vi "Read Message.vi"(8 "error in (no error)":errorcluster, 11 "RemoteControl.ZMQ in":refnum<class "RemoteControl.ZMQ.lvclass">) -> (0 "error out":errorcluster, 1 "Data":string, 2 "Command":string, 3 "RemoteControl.ZMQ out":refnum<class "RemoteControl.ZMQ.lvclass">, 4 "ID":string)   [LabVIEW 2019, in "RemoteControl.ZMQ.lvlib" / "RemoteControl.ZMQ.lvclass"]
uses:
  RemoteControl.ZMQ.lvclass
  <vilib>/addons/zeromq/zmq_socket.lvclass
  <vilib>/addons/zeromq/zmq_context.lvclass
  <vilib>/Utility/error.llb/Error Cluster From Error Code.vi
  <vilib>/ErrorRing/Error Ring.xnode
  <vilib>/PRIrvin/JSON-RPC/JSON-RPC.lvlib
  <userlib>/LevyLab/RemoteControl/RemoteControl/RemoteControl.lvclass
  C:/Program Files (x86)/National Instruments/LabVIEW 2019/user.lib/LevyLab/RemoteControl/RemoteControl/RemoteControl.lvclass
  C:/Program Files (x86)/National Instruments/LabVIEW 2019/vi.lib/JKI/JKI SMO/smo.lvlibp/SMO/SMO.lvclass
panel:
  out "Retry#":i32
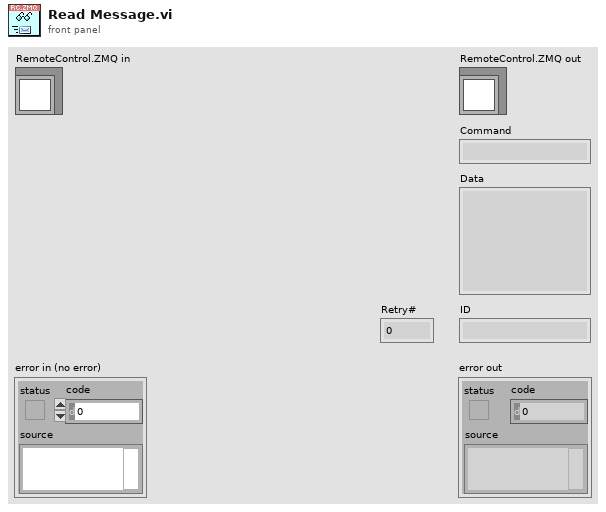
[diagram p1: front panel]
types:
  T1 = typedef "zeromq.lvlib/socket_type.ctl" = enum8{"ZMQ_PAIR", "ZMQ_PUB", "ZMQ_SUB", "ZMQ_REQ", "ZMQ_REP", "ZMQ_DEALER", "ZMQ_ROUTER", "ZMQ_PULL", "ZMQ_PUSH", "ZMQ_XPUB", "ZMQ_XSUB", "ZMQ_STREAM", "ZMQ_SERVER", "ZMQ_CLIENT", "ZMQ_RADIO", "ZMQ_DISH", "ZMQ_GATHER", "ZMQ_SCATTER", "ZMQ_DGRAM"}
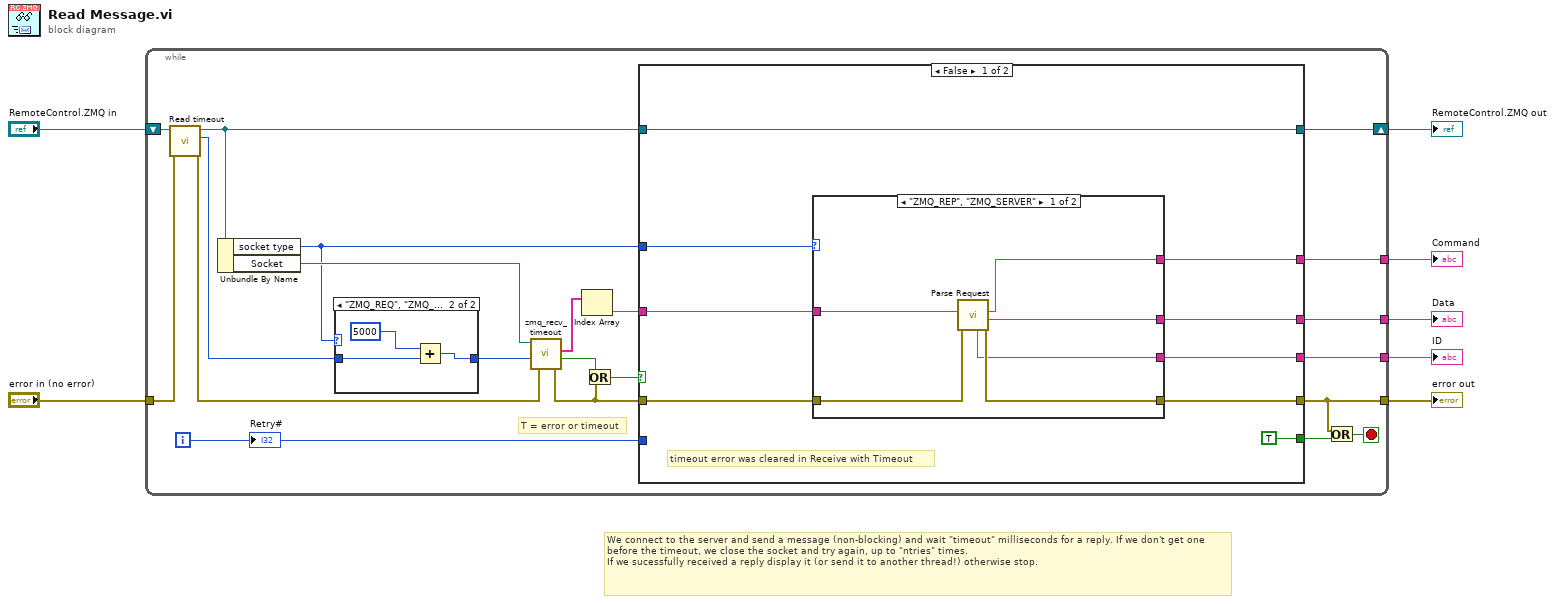
[diagram p0: block diagram]
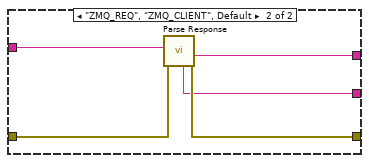
[diagram p3: hidden frame]
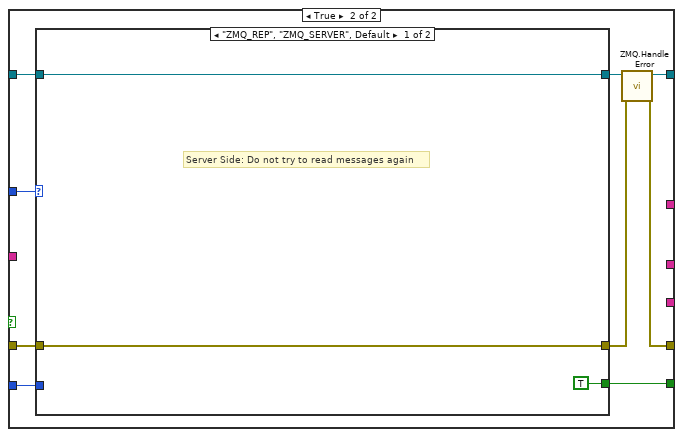
[diagram p4: hidden frame]
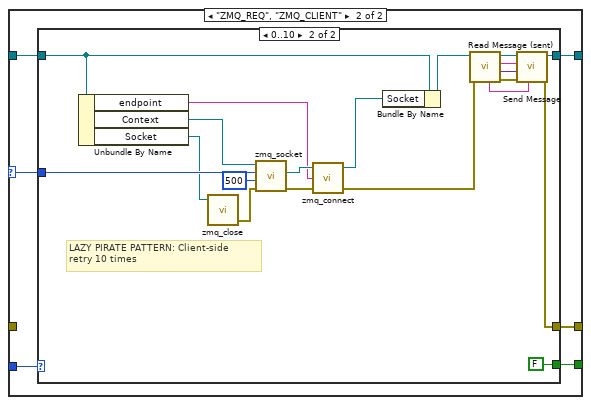
[diagram p5: hidden frame]
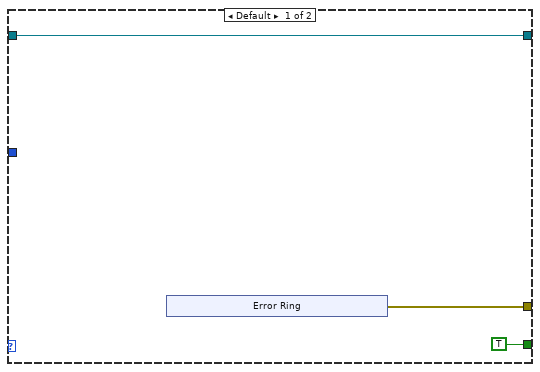
[diagram p6: hidden frame]
diagram:
  # "We connect to the server and send a message (non-blocking) and wait \"timeout\" milliseconds for a reply. If we don't get one before the timeout, we close the socket and try again, up to \"ntries\" times.\nIf we sucessfully received a reply display it (or send it to another thread!) otherwise stop."
  n1 = while {
    tunnel: [w28] -> w7
    tunnel: [w27] -> w6
    tunnel: [w26] -> w5
    tunnel: "error in (no error)" -> [w11]
    tunnel: [w14] -> w4
    shift-right: [w13] -> w3
    shift-left: "RemoteControl.ZMQ in" -> [w12]
    i -> [w23]
    stop <- w25 stop-if-true
    # "T = error or timeout"
    n2 = call <userlib>:"Read timeout.vi"("error in (no error)"=w11, "RemoteControl in"=w12) -> ("error out"=w17:errorcluster, "timeout"=w9:i32, "RemoteControl out"=w16:refnum<class "RemoteControl.ZMQ.lvclass">)  [unwired: 7 in]
    n3 = Unbundle By Name(w16) -> ("socket type"=w10:T1, "Socket"=w18:refnum<class "zmq_socket.lvclass">)
    n4 = case shown="\"ZMQ_REQ\", \"ZMQ_CLIENT\"" w10 {
      tunnel: w9 -> [w29 w32]
      tunnel: [w29 w31] -> w8
      frame "ZMQ_REP", "ZMQ_SERVER", Default {
      }
      frame "ZMQ_REQ", "ZMQ_CLIENT" {
        n5 = Add(x=5000, y=w32) -> (x+y=w31:i32)
      }
    }
    n6 = call <vilib>:"zmq_recv_timeout.vi"("error in"=w17, "timeout (ms)"=w8, "socket in"=w18) -> ("error out"=w21:errorcluster, "timeout?"=w20:bool, "parts"=w15:string[])  [unwired: 1 in, 1 out]
    n7 = Index Array(array=w15) -> (element=w22:string)  [unwired: 1 in]
    n8 = Or(x=w20, y=w21) -> (x .or. y?=w19:bool)
    n9 = case shown="False" w19 {
      tunnel: [w41 _] -> w27
      tunnel: [w40 _] -> w26
      tunnel: [w39 _] -> w28
      tunnel: w10 -> [w38 w60]
      tunnel: w16 -> [w37 w61]
      tunnel: [w37 w53] -> w13
      tunnel: w23 -> [_ w59]
      tunnel: [w36 w54] -> w14
      tunnel: [TRUE w58] -> w24
      tunnel: w21 -> [w35 w57]
      tunnel: w22 -> [w33 _]
      frame False {
        # "timeout error was cleared in Receive with Timeout"
        n10 = case shown="\"ZMQ_REP\", \"ZMQ_SERVER\"" w38 {
          tunnel: w33 -> [w43 w49]
          tunnel: w35 -> [w47 w52]
          tunnel: [w46 w51] -> w36
          tunnel: [w45 _] -> w39
          tunnel: [w42 w48] -> w41
          tunnel: [w44 w50] -> w40
          frame "ZMQ_REP", "ZMQ_SERVER" {
            n11 = call <vilib>:"Parse Request.vi"("error in (no error)"=w47, "<JSON> Requests"=w43) -> ("error out"=w46:errorcluster, "Params"=w42:string, "Methods"=w45:string, "IDs"=w44:string)  [unwired: 6 in]
          }
          frame "ZMQ_REQ", "ZMQ_CLIENT", Default {
            n12 = call <vilib>:"Parse Response.vi"("error in (no error)"=w52, "<JSON> Response"=w49) -> ("error out"=w51:errorcluster, "results"=w48:string, "IDs"=w50:string)  [unwired: 7 in]
          }
        }
      }
      frame True {
        n13 = case shown="\"ZMQ_REP\", \"ZMQ_SERVER\", Default" w60 {
          selector: w60 -> [_ w69]
          tunnel: w61 -> [w64 w70]
          tunnel: [w64 w68] -> w56
          tunnel: w59 -> [_ w65]
          tunnel: [w63 w67] -> w55
          tunnel: [TRUE w66] -> w58
          tunnel: w57 -> [w63 _]
          frame "ZMQ_REP", "ZMQ_SERVER", Default {
            # "Server Side: Do not try to read messages again"
          }
          frame "ZMQ_REQ", "ZMQ_CLIENT" {
            n14 = case shown="0..10" w65 {
              tunnel: w70 -> [w73 w93]
              tunnel: w69 -> [_ w92]
              tunnel: [w73 w86] -> w68
              tunnel: [w72 w80] -> w67
              tunnel: [TRUE FALSE] -> w66
              frame Default {
                n15 = xnode "Error Ring"() -> ("error out"=w72:errorcluster)
              }
              frame 0..10 {
                # "LAZY PIRATE PATTERN: Client-side\nretry 10 times"
                n16 = Unbundle By Name(w93) -> ("endpoint"=w90:string, "Context"=w94:refnum<class "zmq_context.lvclass">, "Socket"=w91:refnum<class "zmq_socket.lvclass">)
                n17 = call <vilib>:"zmq_close.vi"("socket"=w91) -> ("error out"=w97:errorcluster)  [unwired: 4 in]
                n18 = call <vilib>:"zmq_socket.vi"("error in"=w97, "linger (ms)"=500, "socket type"=w92, "context in"=w94) -> ("error out"=w96:errorcluster, "socket out"=w95:refnum<class "zmq_socket.lvclass">)  [unwired: 1 in, 1 out]
                n19 = call <vilib>:"zmq_connect.vi"("error in"=w96, "endpoint"=w90, "socket in"=w95) -> ("error out"=w82:errorcluster, "socket out"=w89:refnum<class "zmq_socket.lvclass">)  [unwired: 1 in]
                n20 = Bundle By Name(cluster=w93, "Socket"=w89) -> (w88:refnum<class "RemoteControl.ZMQ.lvclass">)
                n21 = call <userlib>:"Read Message (sent).vi"("error in (no error)"=w82, "RemoteControl in"=w88) -> ("error out"=w83:errorcluster, "Data (Sent)"=w84:variant, "Command (Sent)"=w85:string, "RemoteControl out"=w87:refnum<class "RemoteControl.ZMQ.lvclass">, "ID (Sent)"=w81:string)  [unwired: 5 in]
                n22 = call-dynamic "Send Message.vi"("ID"=w81, "error in (no error)"=w83, "Data"=w84, "Command"=w85, "RemoteControl.ZMQ in"=w87) -> ("error out"=w80:errorcluster, "RemoteControl.ZMQ out"=w86:refnum<class "RemoteControl.ZMQ.lvclass">)  [unwired: 5 in]
              }
            }
          }
        }
        n23 = call "ZMQ.Handle Error.vi"("error in (no error)"=w55, "RemoteControl.ZMQ in"=w56) -> ("error out"=w54:errorcluster, "RemoteControl.ZMQ out"=w53:refnum<class "RemoteControl.ZMQ.lvclass">)  [unwired: 8 in]
      }
    }
    n24 = Or(x=w14, y=w24) -> (x .or. y?=w25:bool)
    "Retry#" <- w23
  }
  "error out" <- w4
  "RemoteControl.ZMQ out" <- w3
  "ID" <- w5
  "Command" <- w7
  "Data" <- w6
